vi "ULx Get Error Info.vi"(8 "error in":errorcluster, 10 "ErrorCode":i32, 11 "task in":refnum<k24>) -> (0 "error out":errorcluster)   [LabVIEW 2020]
uses:
  C:/Users/William/Documents/LV 2020 builds/LeaktestDAQ/Source-v33/ULx_LV.dll
  ULx_LV.dll
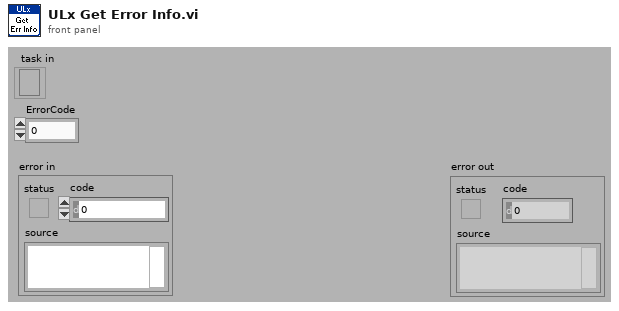
[diagram p1: front panel]
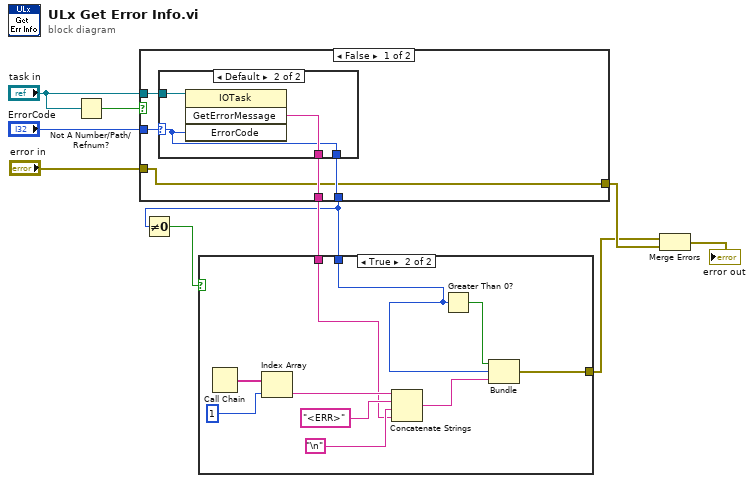
[diagram p0: block diagram]
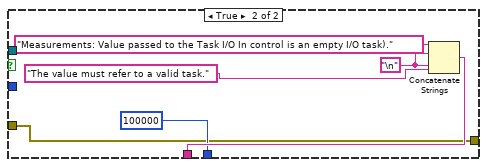
[diagram p4: hidden frame]
diagram:
  n1 = Not A Number/Path/Refnum?(number/path/refnum="task in") -> (NaN/Path/Refnum?=w9:bool)
  n2 = case shown="False" w9 {
    tunnel: [w14 w23] -> w4
    tunnel: [w12 100000] -> w2
    tunnel: "error in" -> [w11 w21]
    tunnel: [w11 w21] -> w8
    tunnel: "task in" -> [w15 _]
    tunnel: "ErrorCode" -> [w13 _]
    frame False {
      n3 = case shown="Default" w13 {
        selector: w13 -> [w16 w17]
        tunnel: w15 -> [_ w19]
        tunnel: [_ w18] -> w14
        tunnel: [w16 w17] -> w12
        frame 0 {
        }
        frame Default {
          n4 = invoke class="IOTask" method="GetErrorMessage"(reference=w19, "ErrorCode"=w17) -> ("GetErrorMessage"=w18:string)  [unwired: 2 in, 3 out]
        }
      }
    }
    frame True {
      w20 = "\n"
      n5 = Concatenate Strings("Measurements: Value passed to the Task I/O In control is an empty I/O task).", w20, w20, "The value must refer to a valid task.") -> (w23:string)
    }
  }
  n6 = Not Equal To 0?(x=w2) -> (x != 0?=w5:bool)
  n7 = case shown="True" w5 {
    tunnel: w4 -> [_ w28]
    tunnel: [_ w27] -> w3
    tunnel: w2 -> [_ w26]
    frame False {
    }
    frame True {
      n8 = Call Chain() -> (call chain=w29:string[])
      n9 = Index Array(array=w29, index=1) -> (element=w31:string)
      n10 = Concatenate Strings(w31, "<ERR>" ("string"), "\n", w28) -> (w32:string)
      n11 = Greater Than 0?(x=w26) -> (x > 0?=w33:bool)
      n12 = Bundle(w33, "ErrorCode"=w26, w32) -> (w27:cluster{bool, "ErrorCode":i32, string})  [unwired: 1 in]
    }
  }
  n13 = Merge Errors(w3, w8) -> (→"error out":errorcluster)
